vi "String_Find Between Tolkens.vi"(6 "Include Dilimeters In Substrings":bool, 7 "Include Dilimeters String":bool, 8 "Second Delimiter":string, 9 "First Delimiter":string, 10 "Seperators {  }":T1, 11 "String":string) -> (0 "Both Dilimeters Found Out":bool, 1 "After Substring Out":string, 2 "Before Substring Out":string, 3 "String Out":string)   [LabVIEW 2020]
uses:
  TypeDefs_Utility/ENUM_String_Between tolkens.ctl
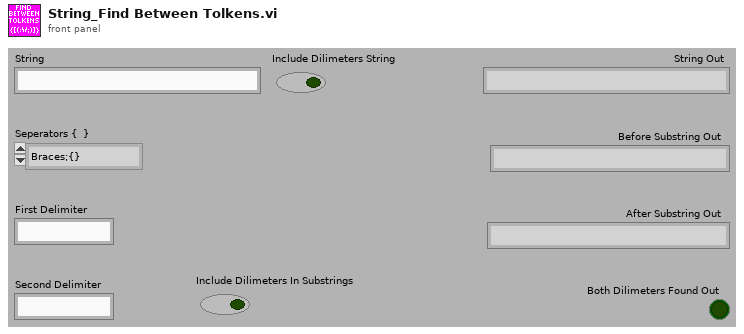
[diagram p1: front panel]
types:
  T1 = typedef "ENUM_String_Between tolkens.ctl" = enum16{"Braces;{}", "Brackets;[]", "Parens;()", "Angles;<>", "Colens;::", "Quotes;\"\"", "Backslashes;\\\\", "None;"}
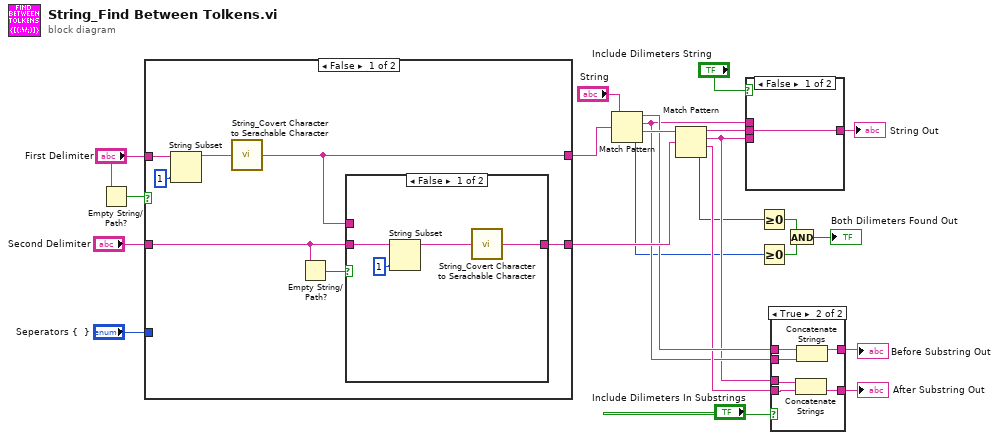
[diagram p0: block diagram]
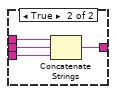
[diagram p2: hidden frame]
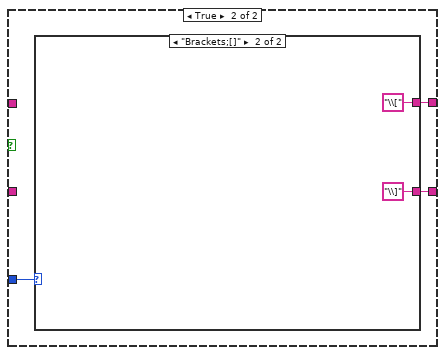
[diagram p5: hidden frame]
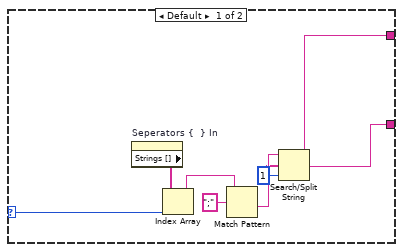
[diagram p6: hidden frame]
diagram:
  n1 = Empty String/Path?(string/path="First Delimiter") -> (empty?=w22:bool)
  n2 = case shown="False" w22 {
    tunnel: "Seperators {  }" -> [_ w36]
    tunnel: [w29 w38] -> w16
    tunnel: [w25 w37] -> w18
    tunnel: "Second Delimiter" -> [w24 _]
    tunnel: "First Delimiter" -> [w28 _]
    frame False {
      n3 = String Subset(string=w28, length (rest)=1 ("length (rest)")) -> (substring=w26:string)  [unwired: 1 in]
      n4 = call "String_Covert Character to Serachable Character.vi"("Char"=w26) -> ("Searchable Char Out"=w25:string)  [unwired: 4 in]
      n5 = Empty String/Path?(string/path=w24) -> (empty?=w30:bool)
      n6 = case shown="False" w30 {
        tunnel: w24 -> [w33 _]
        tunnel: w25 -> [_ w35]
        tunnel: [w31 w35] -> w29
        frame False {
          n7 = String Subset(string=w33, length (rest)=1 ("length (rest)")) -> (substring=w32:string)  [unwired: 1 in]
          n8 = call "String_Covert Character to Serachable Character.vi"("Char"=w32) -> ("Searchable Char Out"=w31:string)  [unwired: 4 in]
        }
        frame True {
        }
      }
    }
    frame True {
      n9 = case shown="\"Brackets;[]\"" w36 {
        selector: w36 -> [w39 _]
        tunnel: [w42 "\\]"] -> w38
        tunnel: [w41 "\\["] -> w37
        frame Default {
          n10 = property on="Seperators {  } In" class="Enum (strict)"() -> ("Strings []"=w40:string[])  [unwired: 2 in, 2 out]
          n11 = Index Array(array=w40, index=w39) -> (element=w46:string)
          n12 = Match Pattern(string=w46, regular expression=";") -> (after substring=w44:string)  [unwired: 1 in, 3 out]
          n13 = Search/Split String(string=w44, offset (0)=1) -> (substring before match=w41:string, match + rest of string=w42:string)  [unwired: 1 in, 1 out]
        }
        frame "Brackets;[]" {
        }
      }
    }
  }
  n14 = Match Pattern(string="String", regular expression=w18) -> (before substring=w15:string, match substring=w7:string, after substring=w17:string, offset past match=w5:i32)  [unwired: 1 in]
  n15 = Match Pattern(string=w17, regular expression=w16) -> (before substring=w8:string, match substring=w6:string, after substring=w12:string, offset past match=w4:i32)  [unwired: 1 in]
  n16 = case shown="False" "Include Dilimeters String" {
    tunnel: w8 -> [w49 w53]
    tunnel: [w49 w52] -> w9
    tunnel: w7 -> [_ w51]
    tunnel: w6 -> [_ w50]
    frame False {
    }
    frame True {
      n17 = Concatenate Strings(w51, w53, w50) -> (w52:string)
    }
  }
  "String Out" <- w9
  n18 = Greater Or Equal To 0?(x=w4) -> (x >= 0?=w2:bool)
  n19 = Greater Or Equal To 0?(x=w5) -> (x >= 0?=w3:bool)
  n20 = case shown="True" "Include Dilimeters In Substrings" {
    tunnel: [w55 w59] -> w14
    tunnel: w15 -> [w55 w61]
    tunnel: w7 -> [_ w58]
    tunnel: w6 -> [_ w56]
    tunnel: w12 -> [w54 w60]
    tunnel: [w54 w57] -> w11
    frame False {
    }
    frame True {
      n21 = Concatenate Strings(w56, w60) -> (w57:string)
      n22 = Concatenate Strings(w61, w58) -> (w59:string)
    }
  }
  "Before Substring Out" <- w14
  "After Substring Out" <- w11
  n23 = And(x=w2, y=w3) -> (x .and. y?=→"Both Dilimeters Found Out":bool)
